vi "Marvin.vi"() -> ()   [LabVIEW 2017]
uses:
  CAN TxRx/CAN/CANalystII/PCAN_Driver/ControlCAN.llb/CAN Channel.ctl
  CAN TxRx/CAN/CANalystII/PCAN_Driver/ControlCAN.llb/DevType.ctl
  CAN TxRx/CAN/CANalystII/PCAN_Driver/ControlCAN.llb/VCI_INIT_CONFIG.ctl
  CAN TxRx/CAN/CANalystII/PCAN_Driver/ControlCAN.llb/InitFlag.ctl
  CAN TxRx/CAN/CANalystII/PCAN_Driver/ControlCAN.llb/Fliter.ctl
  CAN TxRx/CAN/CANalystII/PCAN_Driver/ControlCAN.llb/Mode.ctl
  CAN TxRx/CAN/CANalystII/PCAN_Driver/ControlCAN.llb/VCI_CAN_OBJ.ctl
  CAN TxRx/CAN/CANalystII/PCAN_Driver/ControlCAN.lvlib
panel:
  out "Data Send":u64 format="%016x"
  out "Frame ID":u32=417345319 format="%x"
  in  "Motor Speed RPM":u16
  out "Under voltage/Over voltage":bool
  out "Speed error":bool
  out "Derated drive temp":bool
  out "Motor Over temperature":bool
  out "Commutation err":bool
  out "Motor Sensor temp Fauilre":bool
  out "Drive Over temperature":bool
  out "Drive Sensor temp Failure":bool
  out "Motor Phase Current RMS":dbl
  out "ECS State":u16
  out "Motor Speed RPM":dbl
  out "Motor Stator Temp.":dbl
  out "Power transistor Heat sink Temp.":dbl
  out "DC Current":dbl
  out "DC Voltage":dbl
  out "Array":u64[][](array[numeric]) format="%016x"
  in  "Function":u16(ring) items=["Stop", "Run"]
  in  "Send":bool=TRUE
  out "Date & Time           Frame ID               Length":string
  in  "Stop":bool
  out "Config_CANAT":T7 {"DevType" items=["USB-CAN"=3, "USB-CAN2"=4]; "CanIndex" items=["通道1", "通道2"]; "VCI_INIT_CONFIG"."Fliter" items=["接收所有类型"=3, "只接收标准帧"=4, "只接收扩展帧"=7]; "VCI_INIT_CONFIG"."Mode" items=["正常工作", "自测模式（环回）", "仅侦听模式"]; "VCI_INIT_CONFIG"."InitFlag" items=["使用Flash参数", "使用界面设置参数"]}
  in  "Channel 2":T2 caption="Channel" items=["Channel 1", "Channel 2"]
  out "CAN Statut":bool
  # "ver 1.0"
  # "Marvin"
  # "REDLER TECHNOLOGIES LTD"
  # "0x18E1272F"
  # "0x18E3272F"
  # "0x18E2272F"
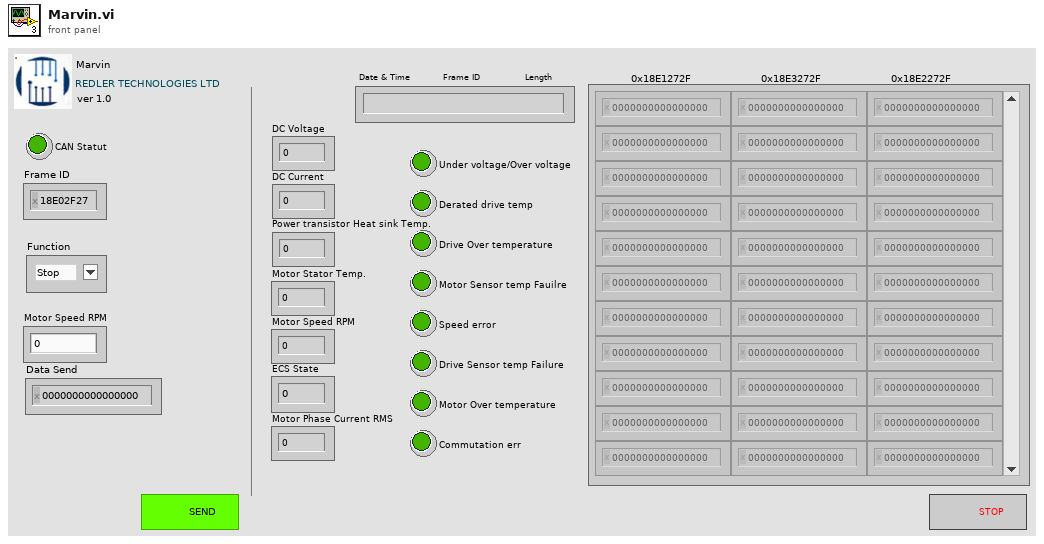
[diagram p1: front panel]
types:
  T1 = typedef "ControlCAN.lvlib/DevType.ctl" = u32
  T2 = typedef "ControlCAN.lvlib/CAN Channel.ctl" = u32
  T3 = typedef "ControlCAN.lvlib/VCI_INIT_CONFIG.ctl" = cluster{"AccCode":u32, "AccMask":u32, "InitFlag":T4, "Fliter":T5, "Timing0":u8, "Timing1":u8, "Mode":T6}
  T4 = typedef "ControlCAN.lvlib/InitFlag.ctl" = u32
  T5 = typedef "ControlCAN.lvlib/Fliter.ctl" = u8
  T6 = typedef "ControlCAN.lvlib/Mode.ctl" = u8
  T7 = cluster{"DevType":T1, "DevIndex":u32, "CanIndex":T2, "VCI_INIT_CONFIG":T3}
  T8 = cluster{"ID":u32, "MSGTYPE":u8, "LEN":u8, "aDATA":u8[]}[]
  T9 = cluster{"ID":u32, "MSGTYPE":u8, "LEN":u8, "aDATA":u8[]}
  T10 = typedef "ControlCAN.lvlib/VCI_CAN_OBJ.ctl" = cluster{"ID":u32, "TimeStamp":u32, "TimeFlag":u8, "SendType":u8, "RemoteFlag":u8, "ExternFlag":u8, "DataLen":u8, "Data":u8[], "Reserved":u8[]}
  T11 = cluster{"Type":enum16{"接收", "发送"}, "Channel":T2, "Time":timestamp, "VCI_CAN_OBJ":T10}[]
  T12 = cluster{"Type":enum16{"接收", "发送"}, "Channel":T2, "Time":timestamp, "VCI_CAN_OBJ":T10}
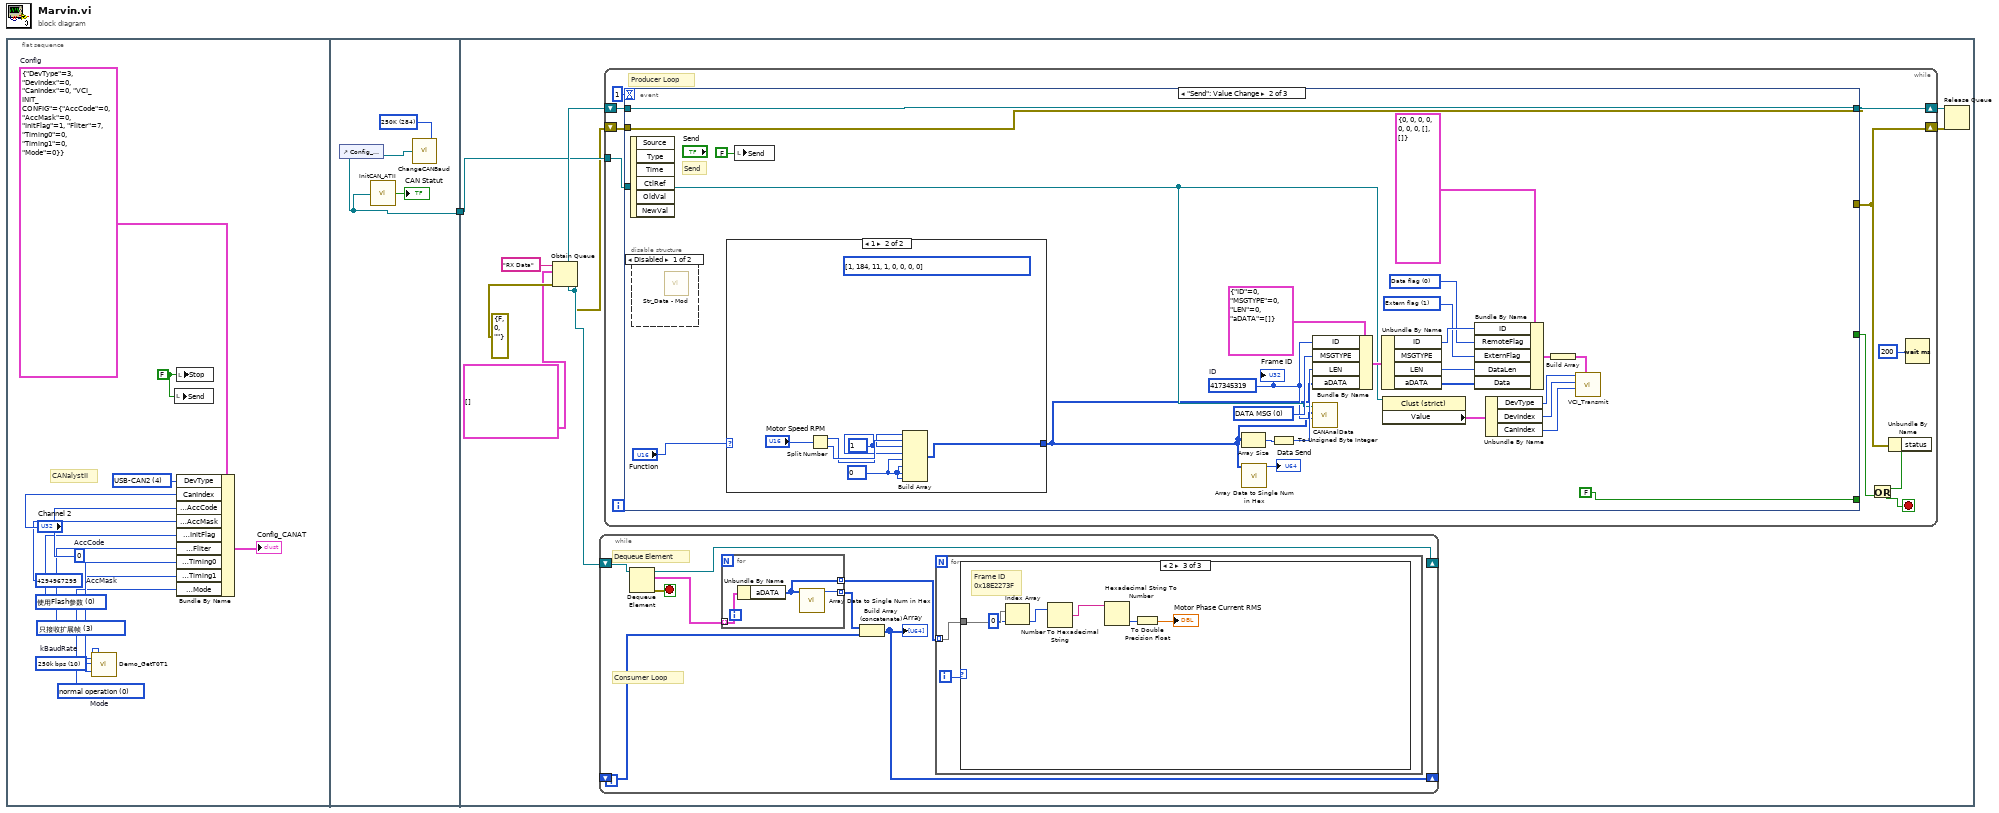
[diagram p0: block diagram]
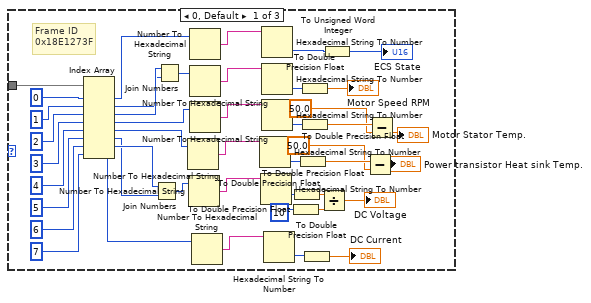
[diagram p2: hidden frame]
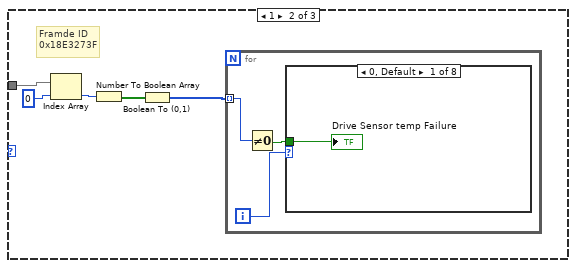
[diagram p3: hidden frame]
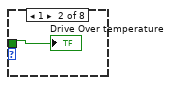
[diagram p4: hidden frame]
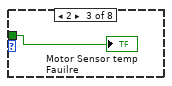
[diagram p5: hidden frame]
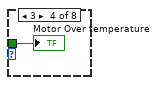
[diagram p6: hidden frame]
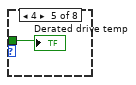
[diagram p7: hidden frame]
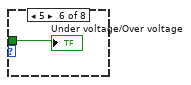
[diagram p8: hidden frame]
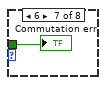
[diagram p9: hidden frame]
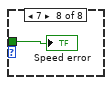
[diagram p10: hidden frame]
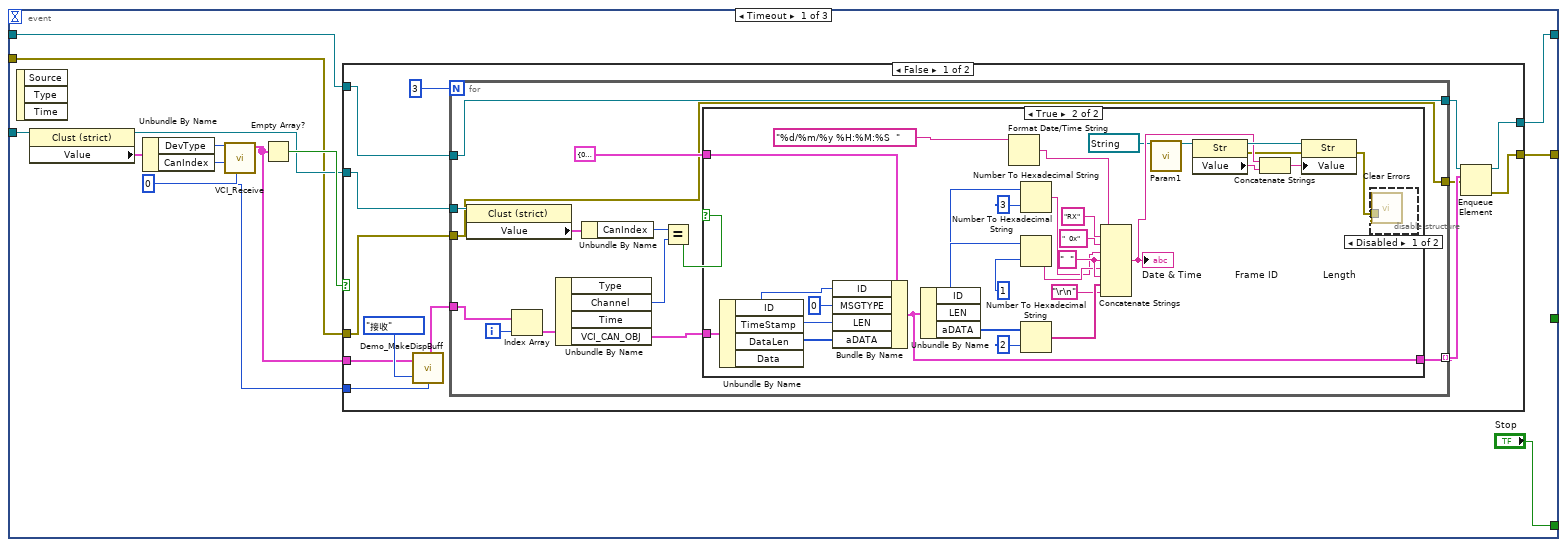
[diagram p11: hidden frame]
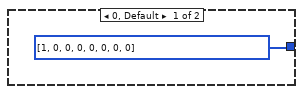
[diagram p15: hidden frame]
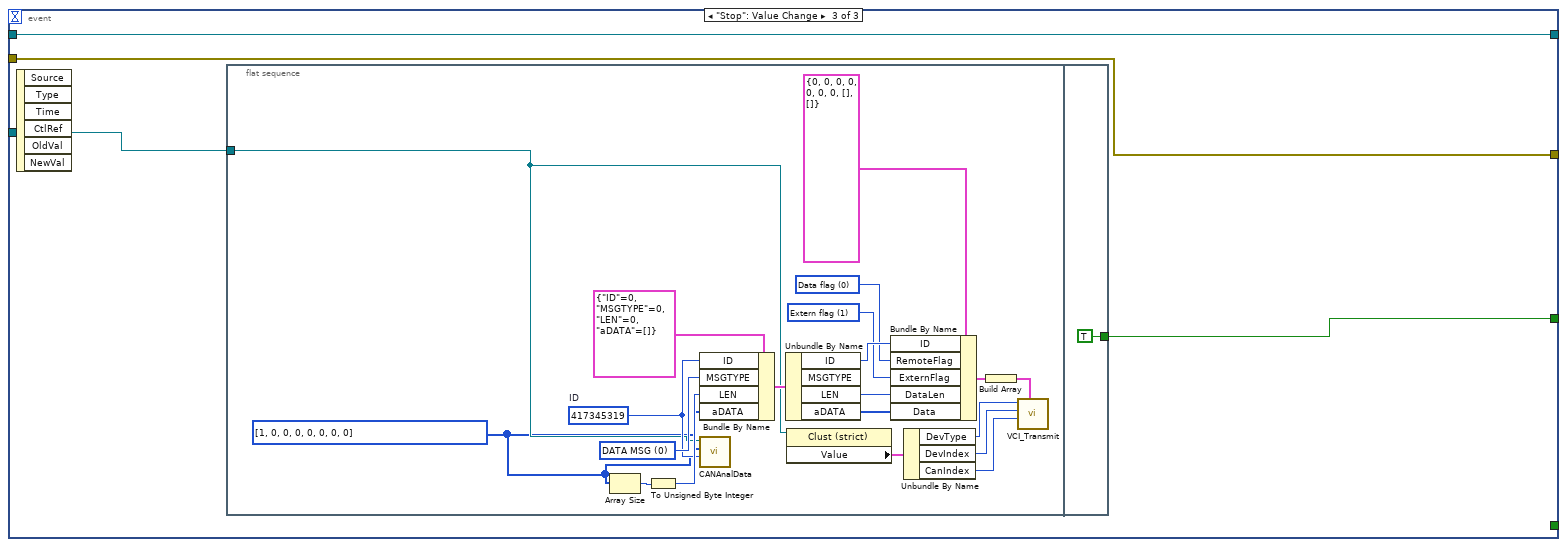
[diagram p17: hidden frame]
diagram:
  n1 = flat-sequence {
    tunnel: [w15] -> w1
    tunnel: w1 -> [w20]
    frame #0 {
      w2 = FALSE ("Stop")
      w10 = u32 4294967295  # AccMask
      w9 = T4 0 items=["使用Flash参数", "使用界面设置参数"] ("InitFlag")
      w4 = T6 0 items=["normal operation", "Listen-only mode", "test mode"]  # Mode
      w8 = T5 3 items=["接收所有类型"=1, "只接收标准帧"=2, "只接收扩展帧"=3] ("Fliter")
      w7 = u8 10 items=["5k bps"=1, "10k bps"=2, "20k bps"=3, "40k bps"=4, "50k bps"=5, "80k bps"=6, "100k bps"=7, "125k bps"=8, "200k bps"=9, "250k bps"=10, "400k bps"=11, "500k bps"=12, "666k bps"=13, "800k bps"=14, "1000k bps"=15, "33.33k bps"=16, "66.66k bps"=17, "83.33k bps"=18]  # kBaudRate
      w11 = u32 0  # AccCode
      w13 = T1 4 items=["USB-CAN"=3, "USB-CAN2"=4] ("DevType")
      w14 = T7 {"DevType"=3, "DevIndex"=0, "CanIndex"=0, "VCI_INIT_CONFIG"={"AccCode"=0, "AccMask"=0, "InitFlag"=1, "Fliter"=7, "Timing0"=0, "Timing1"=0, "Mode"=0}}  # Config
      # "CANalystII"
      n2 = call "Demo_GetT0T1.vi"("kBaudRate"=w7) -> ("Timing0"=w6:u8, "Timing1"=w5:u8)
      n3 = local write "Send"(w2) -> ()
      n4 = local write "Stop"(w2) -> ()
      n5 = Bundle By Name(cluster=w14, "DevType"=w13, "CanIndex"="Channel 2", "VCI_INIT_CONFIG.AccCode"=w11, "VCI_INIT_CONFIG.AccMask"=w10, "VCI_INIT_CONFIG.InitFlag"=w9, "VCI_INIT_CONFIG.Fliter"=w8, "VCI_INIT_CONFIG.Timing0"=w6, "VCI_INIT_CONFIG.Timing1"=w5, "VCI_INIT_CONFIG.Mode"=w4) -> (→"Config_CANAT":T7)
    }
    frame #1 {
      w16 = u16 284 items=["1M"=20, "500K"=28, "250K"=284, "125K"=796, "100K"=17199, "50K"=18223, "20K"=21295, "10K"=26415, "5K"=32639] ("baud in")
      n6 = control-ref of="Config_CANAT"() -> (w15:refnum<vi>)
      n7 = call "InitCAN_ATII.vi"("Config"=w15) -> ("Sts"=→"CAN Statut":bool)
      n8 = call "ChangeCANBaud.vi"("baud in"=w16, "reference"=w15) -> ()
    }
    frame #2 {
      n9 = Obtain Queue(name (unnamed)="RX Data", element data type=T8 [], error in (no error)=errorcluster {"status"=FALSE, "code"=0, "source"=""}) -> (queue out=w21:refnum<queue>, error out=w18:errorcluster)  [unwired: 2 in, 1 out]
      n10 = while {
        shift-right: [w31] -> _
        shift-left: w21 -> [w33]
        shift-right: [w28] -> _
        shift-left: _ -> [w30]
        stop <- w32 stop-if-true
        # "Consumer Loop"
        # "Dequeue Element"
        n11 = Dequeue Element(queue=w33) -> (queue out=w31:refnum<queue>, element=w29:T8, error out=w32:errorcluster)  [unwired: 2 in, 1 out]
        n12 = for {
          tunnel: [w104] -> w27 mode=indexing
          tunnel: w29 -> [w103] mode=indexing
          tunnel: [w102] -> w26 mode=indexing
          n13 = Unbundle By Name(w103) -> ("aDATA"=w102:u8[])
          n14 = call "Array Data to Single Num in Hex.vi"("aDATA"=w102) -> ("Numeric"=w104:u64)  [unwired: 10 in]
        }
        n15 = Build Array (concatenate)(w27, w30) -> (w28:u64[][])
        "Array" <- w28
        n16 = for {
          tunnel: w26 -> [w35] mode=indexing
          i -> [w34]
          n17 = case shown="2" w34 {
            tunnel: w35 -> [w61 w84 w101]
            frame 0, Default {
              # "Frame ID\n0x18E1273F"
              n18 = Index Array(array=w61, index #1=0 ("index"), index #2=1 ("index"), index #3=2 ("index"), index #4=3 ("index"), index #5=4 ("index"), index #6=5 ("index"), index #7=6 ("index"), index #8=7 ("index")) -> (element #1=w44:u8, element #2=w47:u8, element #3=w48:u8, element #4=w52:u8, element #5=w55:u8, element #6=w59:u8, element #7=w60:u8, element #8=w58:u8)
              n19 = Join Numbers(hi=w60, lo=w59) -> ((hi.lo)=w79:u16)
              n20 = Join Numbers(hi=w48, lo=w47) -> ((hi.lo)=w49:u16)
              n21 = Number To Hexadecimal String(2:w55) -> (0:w56:string)  [unwired: 1 in]
              n22 = Number To Hexadecimal String(2:w79) -> (0:w78:string)  [unwired: 1 in]
              n23 = Number To Hexadecimal String(2:w44) -> (0:w45:string)  [unwired: 1 in]
              n24 = Number To Hexadecimal String(2:w49) -> (0:w50:string)  [unwired: 1 in]
              n25 = Number To Hexadecimal String(2:w52) -> (0:w53:string)  [unwired: 1 in]
              n26 = Number To Hexadecimal String(2:w58) -> (0:w72:string)  [unwired: 1 in]
              n27 = Hexadecimal String To Number(string=w56) -> (number=w57:u32)  [unwired: 2 in, 1 out]
              n28 = Hexadecimal String To Number(string=w78) -> (number=w77:u32)  [unwired: 2 in, 1 out]
              n29 = Hexadecimal String To Number(string=w45) -> (number=w42:u32)  [unwired: 2 in, 1 out]
              n30 = Hexadecimal String To Number(string=w50) -> (number=w51:u32)  [unwired: 2 in, 1 out]
              n31 = Hexadecimal String To Number(string=w53) -> (number=w54:u32)  [unwired: 2 in, 1 out]
              n32 = Hexadecimal String To Number(string=w72) -> (number=w71:u32)  [unwired: 2 in, 1 out]
              n33 = To Double Precision Float(number=u32 10 ("y")) -> (double precision float=w75:dbl)
              n34 = To Double Precision Float(number=w77) -> (double precision float=w74:dbl)
              n35 = To Double Precision Float(number=w57) -> (double precision float=w37:dbl)
              n36 = To Double Precision Float(number=w51) -> (double precision float=→"Motor Speed RPM":dbl)
              n37 = To Double Precision Float(number=w54) -> (double precision float=w39:dbl)
              n38 = To Double Precision Float(number=w71) -> (double precision float=→"DC Current":dbl)
              n39 = Divide(x=w74, y=w75) -> (x/y=→"DC Voltage":dbl)
              n40 = To Unsigned Word Integer(number=w42) -> (unsigned 16bit integer=→"ECS State":u16)
              n41 = Subtract(x=w37, y=50.0 ("x")) -> (x-y=→"Power transistor Heat sink Temp.":dbl)
              n42 = Subtract(x=w39, y=50.0 ("x")) -> (x-y=→"Motor Stator Temp.":dbl)
            }
            frame 1 {
              # "Framde ID\n0x18E3273F"
              n43 = Index Array(array=w84, index=0) -> (element=w82:u8)
              n44 = Number To Boolean Array(number=w82) -> (Boolean array=w81:bool[])
              n45 = Boolean To (0,1)(Boolean=w81) -> (0, 1=w80:i16[])
              n46 = for {
                tunnel: w80 -> [w86] mode=indexing
                i -> [w87]
                n47 = Not Equal To 0?(x=w86) -> (x != 0?=w85:bool)
                n48 = case shown="0, Default" w87 {
                  tunnel: w85 -> [w88 w89 w90 w91 w92 w93 w94 w95]
                  frame 0, Default {
                    "Drive Sensor temp Failure" <- w88
                  }
                  frame 1 {
                    "Drive Over temperature" <- w89
                  }
                  frame 2 {
                    "Motor Sensor temp Fauilre" <- w90
                  }
                  frame 3 {
                    "Motor Over temperature" <- w91
                  }
                  frame 4 {
                    "Derated drive temp" <- w92
                  }
                  frame 5 {
                    "Under voltage/Over voltage" <- w93
                  }
                  frame 6 {
                    "Commutation err" <- w94
                  }
                  frame 7 {
                    "Speed error" <- w95
                  }
                }
              }
            }
            frame 2 {
              # "Frame ID\n0x18E2273F"
              n49 = Index Array(array=w101, index=0) -> (element=w98:u8)
              n50 = Number To Hexadecimal String(2:w98) -> (0:w97:string)  [unwired: 1 in]
              n51 = Hexadecimal String To Number(string=w97) -> (number=w99:u32)  [unwired: 2 in, 1 out]
              n52 = To Double Precision Float(number=w99) -> (double precision float=→"Motor Phase Current RMS":dbl)
            }
          }
        }
      }
      n53 = while {
        shift-right: [w108] -> w22
        shift-left: w18 -> [w110]
        shift-right: [w109] -> w23
        shift-left: w21 -> [w111]
        tunnel: w20 -> [w112]
        stop <- w113 stop-if-true
        # "Producer Loop"
        n54 = event shown="[1] \"Send\": Value Change" {
          selector: _ -> [_ _ _]
          dyn-events: _ -> [_ _ _]
          timeout: 1 -> [_ _ _]
          tunnel: ["Stop" FALSE ("Stop") _] -> _
          tunnel: w112 -> [w123 w193 w222]
          tunnel: w111 -> [w119 w213 w224]
          tunnel: w110 -> [w118 w212 w223]
          tunnel: [w116 w213 w224] -> w109
          tunnel: [w115 w212 w223] -> w108
          tunnel: [_ _ w221] -> w105
          event Timeout {
            n55 = event-data() -> ()  [unwired: 1 in, 3 out]
            n56 = property class="Clust (strict)"(reference=w123) -> (reference out=w120:refnum<vi>, "Value"=w124:T7)  [unwired: 1 in, 1 out]
            n57 = Unbundle By Name(w124) -> ("DevType"=w125:T1, "CanIndex"=w121:T2)
            n58 = call "VCI_Receive.vi"("CANIndex"=w121, "DevIndex"=u32 0, "DevType"=w125) -> ("Recieve"=w117:T10[])  [unwired: 3 in, 5 out]
            n59 = Empty Array?(array=w117) -> (empty?=w122:bool)
            n60 = case shown="False" w122 {
              tunnel: w121 -> [w138 _]
              tunnel: w120 -> [w136 _]
              tunnel: w119 -> [w135 w187]
              tunnel: w118 -> [w134 w186]
              tunnel: w117 -> [w139 _]
              tunnel: [w129 w186] -> w115
              tunnel: [w128 w187] -> w116
              frame False {
                n61 = call "Demo_MakeDispBuff.vi"("Channel"=w138, "Type"=enum16{"接收", "发送"}."接收", "OBJs"=w139) -> ("Buffer"=w137:T11)
                n62 = for {
                  N: 3 -> [_]
                  tunnel: w137 -> [w153]
                  tunnel: w136 -> [w152]
                  tunnel: w135 -> [w142]
                  tunnel: w134 -> [w141]
                  tunnel: [w144] -> w132 mode=indexing
                  tunnel: [w142] -> w131
                  tunnel: [w141] -> w130
                  i -> [w145]
                  n63 = property class="Clust (strict)"(reference=w152) -> ("Value"=w150:T7)  [unwired: 1 in, 2 out]
                  n64 = Index Array(array=w153, index=w145) -> (element=w146:T12)
                  n65 = Unbundle By Name(w146) -> ("Channel"=w148:T2, "VCI_CAN_OBJ"=w151:T10)  [unwired: 2 out]
                  n66 = Unbundle By Name(w150) -> ("CanIndex"=w149:T2)
                  n67 = Equal?(x=w149, y=w148) -> (x = y?=w147:bool)
                  n68 = case shown="True" w147 {
                    tunnel: w151 -> [_ w184]
                    tunnel: [w154 w156] -> w144
                    tunnel: T9 {"ID"=0, "MSGTYPE"=0, "LEN"=0, "aDATA"=[]} ("Msg") -> [w154 w155]
                    frame False {
                    }
                    frame True {
                      w169 = "  " ("string")
                      n69 = Unbundle By Name(w184) -> ("ID"=w183:u32, "DataLen"=w182:u8, "Data"=w157:u8[])  [unwired: 1 out]
                      n70 = Bundle By Name(cluster=w155, "ID"=w183, "MSGTYPE"=u8 0, "LEN"=w182, "aDATA"=w157) -> (w156:T9)
                      n71 = Unbundle By Name(w156) -> ("ID"=w162:u32, "LEN"=w163:u8, "aDATA"=w170:u8[])
                      n72 = Format Date/Time String(time format string (%c)="%d/%m/%y %H:%M:%S  ") -> (date/time string=w180:string)  [unwired: 2 in]
                      n73 = Number To Hexadecimal String(1:i16 3 ("width (-)"), 2:w162) -> (0:w167:string)
                      n74 = Number To Hexadecimal String(1:i16 1 ("width (-)"), 2:w163) -> (0:w168:string)
                      n75 = Number To Hexadecimal String(1:i16 2 ("width (-)"), 2:w170) -> (0:w171:string[])
                      n76 = Concatenate Strings(w180, "RX" ("string"), "  0x" ("string"), w167, w169, w168, w169, w171, "\r\n") -> (w173:string)
                      "Date & Time           Frame ID               Length" <- w173
                      n77 = call "Param1.vi"("str"=refnum<vi> refnum) -> ("str out"=w174:refnum<vi>)  [unwired: 17 in, 1 out]
                      n78 = property class="Str"(reference=w174) -> (reference out=w176:refnum<vi>, error out=w159:errorcluster, "Value"=w177:string)  [unwired: 1 in]
                      n79 = Concatenate Strings(w173, w177) -> (w175:string)
                      n80 = property class="Str"(reference=w176, error in=w159, "Value"=w175) -> (error out=w158:errorcluster)  [unwired: 1 out]
                      n81 = disable-structure shown="Disabled" {
                        disable-tunnel: w158 -> [w185 _]
                        frame Disabled {
                          n82 = call <vilib>:"Clear Errors.vi"("error in (no error)"=w185) -> ()  [unwired: 5 in, 2 out]
                        }
                        frame Enabled {
                        }
                      }
                    }
                  }
                }
                n83 = Enqueue Element(queue=w131, element=w132, error in (no error)=w130) -> (queue out=w128:refnum<queue>, error out=w129:errorcluster)  [unwired: 2 out]
              }
              frame True {
              }
            }
          }
          event "Send": Value Change {
            w195 = u8 0 items=["STATUS"=128, "EXTENDED"=2, "RTR"=1, "DATA MSG"=0] ("MSGTYPE")
            w200 = u8 1 items=["Standart flag", "Extern flag"] ("Format")
            w199 = u8 0 items=["Data flag", "Remote flag"] ("Type")
            w192 = u32 417345319  # ID
            # "Send"
            n84 = event-data() -> ()  [unwired: 1 in, 6 out]
            n85 = disable-structure shown="Disabled" {
              frame Disabled {
                n86 = call "Str_Data - Mod.vi"() -> ()  [unwired: 6 in, 1 out]
              }
              frame Enabled {
              }
            }
            n87 = case shown="1" "Function" {
              tunnel: [u8[] [1, 0, 0, 0, 0, 0, 0, 0] ("Data 2") w215] -> w189
              frame 0, Default {
              }
              frame 1 {
                w216 = u8 0 ("element")
                w217 = u8 1 ("element")
                (unwired) u8[] [1, 184, 11, 1, 0, 0, 0, 0] ("Data 2")
                n88 = Split Number(x="Motor Speed RPM") -> (hi(x)=w218:u8, lo(x)=w219:u8)
                n89 = Build Array(w217, w219, w218, w217, w216, w216, w216, w216) -> (w215:u8[])
              }
            }
            n90 = local write "Send"(FALSE ("Send")) -> ()
            n91 = Array Size(array=w189) -> (size(s)=w198:i32)
            n92 = call "Array Data to Single Num in Hex.vi"("aDATA"=w189) -> ("Numeric"=→"Data Send":u64)  [unwired: 10 in]
            n93 = To Unsigned Byte Integer(number=w198) -> (unsigned 8bit integer=w196:u8)
            n94 = Bundle By Name(cluster=T9 {"ID"=0, "MSGTYPE"=0, "LEN"=0, "aDATA"=[]} ("MsgTX 2"), "ID"=w192, "MSGTYPE"=w195, "LEN"=w196, "aDATA"=w189) -> (w194:T9)
            n95 = call "CANAnalData.vi"("ID"=w192, "Data"=w189, "Config"=w193) -> ()  [unwired: 4 in, 5 out]
            n96 = Unbundle By Name(w194) -> ("ID"=w208:u32, "LEN"=w209:u8, "aDATA"=w210:u8[])  [unwired: 1 out]
            n97 = property class="Clust (strict)"(reference=w193) -> ("Value"=w207:T7)  [unwired: 1 in, 2 out]
            n98 = Bundle By Name(cluster=T10 {"ID"=0, "TimeStamp"=0, "TimeFlag"=0, "SendType"=0, "RemoteFlag"=0, "ExternFlag"=0, "DataLen"=0, "Data"=[], "Reserved"=[]} ("Send"), "ID"=w208, "RemoteFlag"=w199, "ExternFlag"=w200, "DataLen"=w209, "Data"=w210) -> (w205:T10)
            n99 = Unbundle By Name(w207) -> ("DevType"=w201:T1, "DevIndex"=w202:u32, "CanIndex"=w203:T2)
            n100 = Build Array(w205) -> (w204:T10[])
            n101 = call "VCI_Transmit.vi"("Buffer"=w204, "CANIndex"=w203, "DevIndex"=w202, "DevType"=w201) -> ()  [unwired: 1 in, 7 out]
            "Frame ID" <- w192
          }
          event "Stop": Value Change {
            n102 = event-data() -> ()  [unwired: 1 in, 6 out]
            n103 = flat-sequence {
              tunnel: w222 -> [w226]
              tunnel: [TRUE ("Stop")] -> w221
              frame #0 {
                w225 = u8[] [1, 0, 0, 0, 0, 0, 0, 0] ("Data 2")
                w229 = u8 0 items=["STATUS"=128, "EXTENDED"=2, "RTR"=1, "DATA MSG"=0] ("MSGTYPE")
                w234 = u8 1 items=["Standart flag", "Extern flag"] ("Format")
                w233 = u8 0 items=["Data flag", "Remote flag"] ("Type")
                w227 = u32 417345319  # ID
                n104 = Array Size(array=w225) -> (size(s)=w232:i32)
                n105 = To Unsigned Byte Integer(number=w232) -> (unsigned 8bit integer=w230:u8)
                n106 = Bundle By Name(cluster=T9 {"ID"=0, "MSGTYPE"=0, "LEN"=0, "aDATA"=[]} ("MsgTX 2"), "ID"=w227, "MSGTYPE"=w229, "LEN"=w230, "aDATA"=w225) -> (w228:T9)
                n107 = call "CANAnalData.vi"("ID"=w227, "Data"=w225, "Config"=w226) -> ()  [unwired: 4 in, 5 out]
                n108 = Unbundle By Name(w228) -> ("ID"=w242:u32, "LEN"=w243:u8, "aDATA"=w244:u8[])  [unwired: 1 out]
                n109 = property class="Clust (strict)"(reference=w226) -> ("Value"=w241:T7)  [unwired: 1 in, 2 out]
                n110 = Bundle By Name(cluster=T10 {"ID"=0, "TimeStamp"=0, "TimeFlag"=0, "SendType"=0, "RemoteFlag"=0, "ExternFlag"=0, "DataLen"=0, "Data"=[], "Reserved"=[]} ("Send"), "ID"=w242, "RemoteFlag"=w233, "ExternFlag"=w234, "DataLen"=w243, "Data"=w244) -> (w239:T10)
                n111 = Unbundle By Name(w241) -> ("DevType"=w235:T1, "DevIndex"=w236:u32, "CanIndex"=w237:T2)
                n112 = Build Array(w239) -> (w238:T10[])
                n113 = call "VCI_Transmit.vi"("Buffer"=w238, "CANIndex"=w237, "DevIndex"=w236, "DevType"=w235) -> ()  [unwired: 1 in, 7 out]
              }
              frame #1 {
              }
            }
          }
        }
        n114 = Unbundle By Name(w108) -> ("status"=w114:bool)
        n115 = Or(x=w114, y=w105) -> (x .or. y?=w113:bool)
        n116 = Wait (ms)(milliseconds to wait=u32 200) -> ()  [unwired: 1 out]
      }
      n117 = Release Queue(queue=w23, error in (no error)=w22) -> ()  [unwired: 1 in, 3 out]
    }
  }
